vi "Read Autonomous.vi"() -> ()   [LabVIEW 2011]
uses:
  Shared/Autonomous Recording TypeDef.ctl
panel:
  out "Array":T1[](array[typedef])
  in  "Path":path
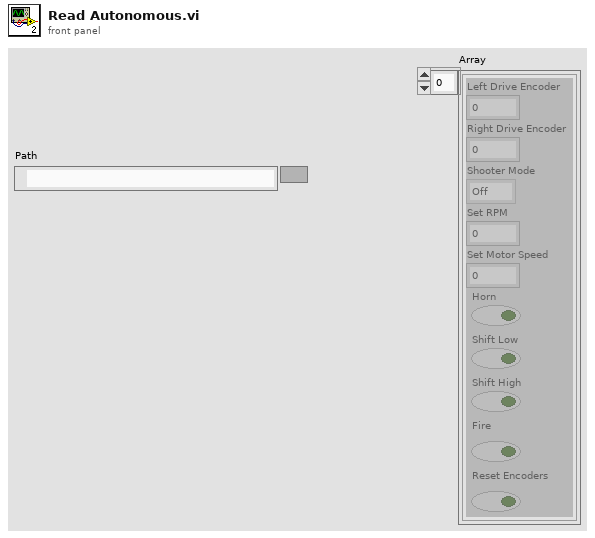
[diagram p1: front panel]
types:
  T1 = typedef "Autonomous Recording TypeDef.ctl" = cluster{"Left Drive Encoder":dbl, "Right Drive Encoder":dbl, "Shooter Mode":enum16{"Off", "Open Loop Control", "Closed Loop Control", "Top Spin"}, "Set RPM":dbl, "Set Motor Speed":dbl, "Horn":bool, "Shift Low":bool, "Shift High":bool, "Fire":bool, "Reset Encoders":bool}
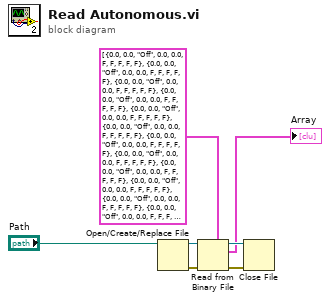
[diagram p0: block diagram]
diagram:
  n1 = Open/Create/Replace File(file path (use dialog)="Path") -> (refnum out=w6:refnum<file>, error out=w7:errorcluster)  [unwired: 5 in, 1 out]
  n2 = Read from Binary File(5:T1[] [{"Left Drive Encoder"=0.0, "Right Drive Encoder"=0.0, "Shooter Mode"=enum."Off", "Set RPM"=0.0, "Set Motor Speed"=0.0, "Horn"=FALSE, "Shift Low"=FALSE, "Shift High"=FALSE, "Fire"=FALSE, "Reset Encoders"=FALSE}, {"Left Drive Encoder"=0.0, "Right Drive Encoder"=0.0, "Shooter Mode"=enum."Off", "Set RPM"=0.0, "Set Motor Speed"=0.0, "Horn"=FALSE, "Shift Low"=FALSE, "Shift High"=FALSE, "Fire"=FALSE, "Reset Encoders"=FALSE}, {"Left Drive Encoder"=0.0, "Right Drive Encoder"=0.0, "Shooter Mode"=enum."Off", "Set RPM"=0.0, "Set Motor Speed"=0.0, "Horn"=FALSE, "Shift Low"=FALSE, "Shift High"=FALSE, "Fire"=FALSE, "Reset Encoders"=FALSE}, {"Left Drive Encoder"=0.0, "Right Drive Encoder"=0.0, "Shooter Mode"=enum."Off", "Set RPM"=0.0, "Set Motor Speed"=0.0, "Horn"=FALSE, "Shift Low"=FALSE, "Shift High"=FALSE, "Fire"=FALSE, "Reset Encoders"=FALSE}, {"Left Drive Encoder"=0.0, "Right Drive Encoder"=0.0, "Shooter Mode"=enum."Off", "Set RPM"=0.0, "Set Motor Speed"=0.0, "Horn"=FALSE, "Shift Low"=FALSE, "Shift High"=FALSE, "Fire"=FALSE, "Reset Encoders"=FALSE}, {"Left Drive Encoder"=0.0, "Right Drive Encoder"=0.0, "Shooter Mode"=enum."Off", "Set RPM"=0.0, "Set Motor Speed"=0.0, "Horn"=FALSE, "Shift Low"=FALSE, "Shift High"=FALSE, "Fire"=FALSE, "Reset Encoders"=FALSE}, {"Left Drive Encoder"=0.0, "Right Drive Encoder"=0.0, "Shooter Mode"=enum."Off", "Set RPM"=0.0, "Set Motor Speed"=0.0, "Horn"=FALSE, "Shift Low"=FALSE, "Shift High"=FALSE, "Fire"=FALSE, "Reset Encoders"=FALSE}, {"Left Drive Encoder"=0.0, "Right Drive Encoder"=0.0, "Shooter Mode"=enum."Off", "Set RPM"=0.0, "Set Motor Speed"=0.0, "Horn"=FALSE, "Shift Low"=FALSE, "Shift High"=FALSE, "Fire"=FALSE, "Reset Encoders"=FALSE}, {"Left Drive Encoder"=0.0, "Right Drive Encoder"=0.0, "Shooter Mode"=enum."Off", "Set RPM"=0.0, "Set Motor Speed"=0.0, "Horn"=FALSE, "Shift Low"=FALSE, "Shift High"=FALSE, "Fire"=FALSE, "Reset Encoders"=FALSE}, {"Left Drive Encoder"=0.0, "Right Drive Encoder"=0.0, "Shooter Mode"=enum."Off", "Set RPM"=0.0, "Set Motor Speed"=0.0, "Horn"=FALSE, "Shift Low"=FALSE, "Shift High"=FALSE, "Fire"=FALSE, "Reset Encoders"=FALSE}, {"Left Drive Encoder"=0.0, "Right Drive Encoder"=0.0, "Shooter Mode"=enum."Off", "Set RPM"=0.0, "Set Motor Speed"=0.0, "Horn"=FALSE, "Shift Low"=FALSE, "Shift High"=FALSE, "Fire"=FALSE, "Reset Encoders"=FALSE}, {"Left Drive Encoder"=0.0, "Right Drive Encoder"=0.0, "Shooter Mode"=enum."Off", "Set RPM"=0.0, "Set Motor Speed"=0.0, "Horn"=FALSE, "Shift Low"=FALSE, "Shift High"=FALSE, "Fire"=FALSE, "Reset Encoders"=FALSE}, {"Left Drive Encoder"=0.0, "Right Drive Encoder"=0.0, "Shooter Mode"=enum."Off", "Set RPM"=0.0, "Set Motor Speed"=0.0, "Horn"=FALSE, "Shift Low"=FALSE, "Shift High"=FALSE, "Fire"=FALSE, "Reset Encoders"=FALSE}, {"Left Drive Encoder"=0.0, "Right Drive Encoder"=0.0, "Shooter Mode"=enum."Off", "Set RPM"=0.0, "Set Motor Speed"=0.0, "Horn"=FALSE, "Shift Low"=FALSE, "Shift High"=FALSE, "Fire"=FALSE, "Reset Encoders"=FALSE}, {"Left Drive Encoder"=0.0, "Right Drive Encoder"=0.0, "Shooter Mode"=enum."Off", "Set RPM"=0.0, "Set Motor Speed"=0.0, "Horn"=FALSE, "Shift Low"=FALSE, "Shift High"=FALSE, "Fire"=FALSE, "Reset Encoders"=FALSE}, {"Left Drive Encoder"=0.0, "Right Drive Encoder"=0.0, "Shooter Mode"=enum."Off", "Set RPM"=0.0, "Set Motor Speed"=0.0, "Horn"=FALSE, "Shift Low"=FALSE, "Shift High"=FALSE, "Fire"=FALSE, "Reset Encoders"=FALSE}, {"Left Drive Encoder"=0.0, "Right Drive Encoder"=0.0, "Shooter Mode"=enum."Off", "Set RPM"=0.0, "Set Motor Speed"=0.0, "Horn"=FALSE, "Shift Low"=FALSE, "Shift High"=FALSE, "Fire"=FALSE, "Reset Encoders"=FALSE}, {"Left Drive Encoder"=0.0, "Right Drive Encoder"=0.0, "Shooter Mode"=enum."Off", "Set RPM"=0.0, "Set Motor Speed"=0.0, "Horn"=FALSE, "Shift Low"=FALSE, "Shift High"=FALSE, "Fire"=FALSE, "Reset Encoders"=FALSE}, {"Left Drive Encoder"=0.0, "Right Drive Encoder"=0.0, "Shooter Mode"=enum."Off", "Set RPM"=0.0, "Set Motor Speed"=0.0, "Horn"=FALSE, "Shift Low"=FALSE, "Shift High"=FALSE, "Fire"=FALSE, "Reset Encoders"=FALSE}, {"Left Drive Encoder"=0.0, "Right Drive Encoder"=0.0, "Shooter Mode"=enum."Off", "Set RPM"=0.0, "Set Motor Speed"=0.0, "Horn"=FALSE, "Shift Low"=FALSE, "Shift High"=FALSE, "Fire"=FALSE, "Reset Encoders"=FALSE}, {"Left Drive Encoder"=0.0, "Right Drive Encoder"=0.0, "Shooter Mode"=enum."Off", "Set RPM"=0.0, "Set Motor Speed"=0.0, "Horn"=FALSE, "Shift Low"=FALSE, "Shift High"=FALSE, "Fire"=FALSE, "Reset Encoders"=FALSE}, {"Left Drive Encoder"=0.0, "Right Drive Encoder"=0.0, "Shooter Mode"=enum."Off", "Set RPM"=0.0, "Set Motor Speed"=0.0, "Horn"=FALSE, "Shift Low"=FALSE, "Shift High"=FALSE, "Fire"=FALSE, "Reset Encoders"=FALSE}, {"Left Drive Encoder"=0.0, "Right Drive Encoder"=0.0, "Shooter Mode"=enum."Off", "Set RPM"=0.0, "Set Motor Speed"=0.0, "Horn"=FALSE, "Shift Low"=FALSE, "Shift High"=FALSE, "Fire"=FALSE, "Reset Encoders"=FALSE}, {"Left Drive Encoder"=0.0, "Right Drive Encoder"=0.0, "Shooter Mode"=enum."Off", "Set RPM"=0.0, "Set Motor Speed"=0.0, "Horn"=FALSE, "Shift Low"=FALSE, "Shift High"=FALSE, "Fire"=FALSE, "Reset Encoders"=FALSE}, {"Left Drive Encoder"=0.0, "Right Drive Encoder"=0.0, "Shooter Mode"=enum."Off", "Set RPM"=0.0, "Set Motor Speed"=0.0, "Horn"=FALSE, "Shift Low"=FALSE, "Shift High"=FALSE, "Fire"=FALSE, "Reset Encoders"=FALSE}, {"Left Drive Encoder"=0.0, "Right Drive Encoder"=0.0, "Shooter Mode"=enum."Off", "Set RPM"=0.0, "Set Motor Speed"=0.0, "Horn"=FALSE, "Shift Low"=FALSE, "Shift High"=FALSE, "Fire"=FALSE, "Reset Encoders"=FALSE}, {"Left Drive Encoder"=0.0, "Right Drive Encoder"=0.0, "Shooter Mode"=enum."Off", "Set RPM"=0.0, "Set Motor Speed"=0.0, "Horn"=FALSE, "Shift Low"=FALSE, "Shift High"=FALSE, "Fire"=FALSE, "Reset Encoders"=FALSE}, {"Left Drive Encoder"=0.0, "Right Drive Encoder"=0.0, "Shooter Mode"=enum."Off", "Set RPM"=0.0, "Set Motor Speed"=0.0, "Horn"=FALSE, "Shift Low"=FALSE, "Shift High"=FALSE, "Fire"=FALSE, "Reset Encoders"=FALSE}, {"Left Drive Encoder"=0.0, "Right Drive Encoder"=0.0, "Shooter Mode"=enum."Off", "Set RPM"=0.0, "Set Motor Speed"=0.0, "Horn"=FALSE, "Shift Low"=FALSE, "Shift High"=FALSE, "Fire"=FALSE, "Reset Encoders"=FALSE}, {"Left Drive Encoder"=0.0, "Right Drive Encoder"=0.0, "Shooter Mode"=enum."Off", "Set RPM"=0.0, "Set Motor Speed"=0.0, "Horn"=FALSE, "Shift Low"=FALSE, "Shift High"=FALSE, "Fire"=FALSE, "Reset Encoders"=FALSE}, {"Left Drive Encoder"=0.0, "Right Drive Encoder"=0.0, "Shooter Mode"=enum."Off", "Set RPM"=0.0, "Set Motor Speed"=0.0, "Horn"=FALSE, "Shift Low"=FALSE, "Shift High"=FALSE, "Fire"=FALSE, "Reset Encoders"=FALSE}, {"Left Drive Encoder"=0.0, "Right Drive Encoder"=0.0, "Shooter Mode"=enum."Off", "Set RPM"=0.0, "Set Motor Speed"=0.0, "Horn"=FALSE, "Shift Low"=FALSE, "Shift High"=FALSE, "Fire"=FALSE, "Reset Encoders"=FALSE}, {"Left Drive Encoder"=0.0, "Right Drive Encoder"=0.0, "Shooter Mode"=enum."Off", "Set RPM"=0.0, "Set Motor Speed"=0.0, "Horn"=FALSE, "Shift Low"=FALSE, "Shift High"=FALSE, "Fire"=FALSE, "Reset Encoders"=FALSE}, {"Left Drive Encoder"=0.0, "Right Drive Encoder"=0.0, "Shooter Mode"=enum."Off", "Set RPM"=0.0, "Set Motor Speed"=0.0, "Horn"=FALSE, "Shift Low"=FALSE, "Shift High"=FALSE, "Fire"=FALSE, "Reset Encoders"=FALSE}, {"Left Drive Encoder"=0.0, "Right Drive Encoder"=0.0, "Shooter Mode"=enum."Off", "Set RPM"=0.0, "Set Motor Speed"=0.0, "Horn"=FALSE, "Shift Low"=FALSE, "Shift High"=FALSE, "Fire"=FALSE, "Reset Encoders"=FALSE}, {"Left Drive Encoder"=-1.7999999999999998, "Right Drive Encoder"=-1.7999999999999998, "Shooter Mode"=enum."Off", "Set RPM"=0.0, "Set Motor Speed"=0.0, "Horn"=FALSE, "Shift Low"=FALSE, "Shift High"=FALSE, "Fire"=FALSE, "Reset Encoders"=FALSE}, {"Left Drive Encoder"=-8.64, "Right Drive Encoder"=-6.12, "Shooter Mode"=enum."Off", "Set RPM"=0.0, "Set Motor Speed"=0.0, "Horn"=FALSE, "Shift Low"=FALSE, "Shift High"=FALSE, "Fire"=FALSE, "Reset Encoders"=FALSE}, {"Left Drive Encoder"=-14.399999999999999, "Right Drive Encoder"=-13.68, "Shooter Mode"=enum."Off", "Set RPM"=0.0, "Set Motor Speed"=0.0, "Horn"=FALSE, "Shift Low"=FALSE, "Shift High"=FALSE, "Fire"=FALSE, "Reset Encoders"=FALSE}, {"Left Drive Encoder"=-24.119999999999997, "Right Drive Encoder"=-27.36, "Shooter Mode"=enum."Off", "Set RPM"=0.0, "Set Motor Speed"=0.0, "Horn"=FALSE, "Shift Low"=FALSE, "Shift High"=FALSE, "Fire"=FALSE, "Reset Encoders"=FALSE}, {"Left Drive Encoder"=-36.36, "Right Drive Encoder"=0.0, "Shooter Mode"=enum."Off", "Set RPM"=0.0, "Set Motor Speed"=0.0, "Horn"=FALSE, "Shift Low"=FALSE, "Shift High"=FALSE, "Fire"=FALSE, "Reset Encoders"=FALSE}] ("Array"), 8:w7, 11:w6) -> (0:w3:errorcluster, 2:→"Array":T1[], 3:w4:refnum<file>)  [unwired: 3 in, 1 out]
  n3 = Close File(refnum=w4, error in=w3) -> ()  [unwired: 2 out]
